vi "FPGAcode2.1.vi"() -> ()   [LabVIEW 2015]
uses:
  Detector_Cluster.ctl
  Limits_In.ctl
  <vilib>/Platform/TimedLoop/XDataNode/timing_clust.ctl
  <vilib>/Platform/TimedLoop/XDataNode/nitl_modes.ctl
  <vilib>/Platform/TimedLoop/XDataNode/wakeup.ctl
  <vilib>/rvi/Emulation/niFpgaSctlEmulationGetInTimedLoop.vi
  <vilib>/rvi/Emulation/niFpgaEmulationReportErrorSimple.vi
  <vilib>/rvi/Emulation/niFpgaGetClockAttributes.vi
  <vilib>/rvi/Emulation/niFpgaCriticalErrorInLSC.vi
  <vilib>/rvi/Emulation/niFpgaProcessEmulError.vi
  <vilib>/rvi/eio/common/nirviEmuTemplateMethod_errors.vi
  <vilib>/Platform/TimedLoop/XDataNode/XDataNode.xnode
  <vilib>/eio/EIONode/EIONode.xnode
  <vilib>/Platform/TimedLoop/XDataNode/XDNodeRunTimeDep.lvlib
panel:
  in  "Limits":T1
  in  "Filter Thresholds":T2
  out "Detector 3 Max Correlations":T2
  out "Detector 3 Correlations":T2
  out "Detector 1 Correlations":T2
  in  "Calibrate":bool
  out "IO Module\\AI 1":i16
  out "IO Module\\AI 0":i16
  out "Del Armed":bool
  out "Armed":bool
  out "Delay":bool
  out "Plates":bool
  in  "Reset One Shot":bool
  in  "One Shot":bool
  in  "Mult1":fxp<+,16,7>
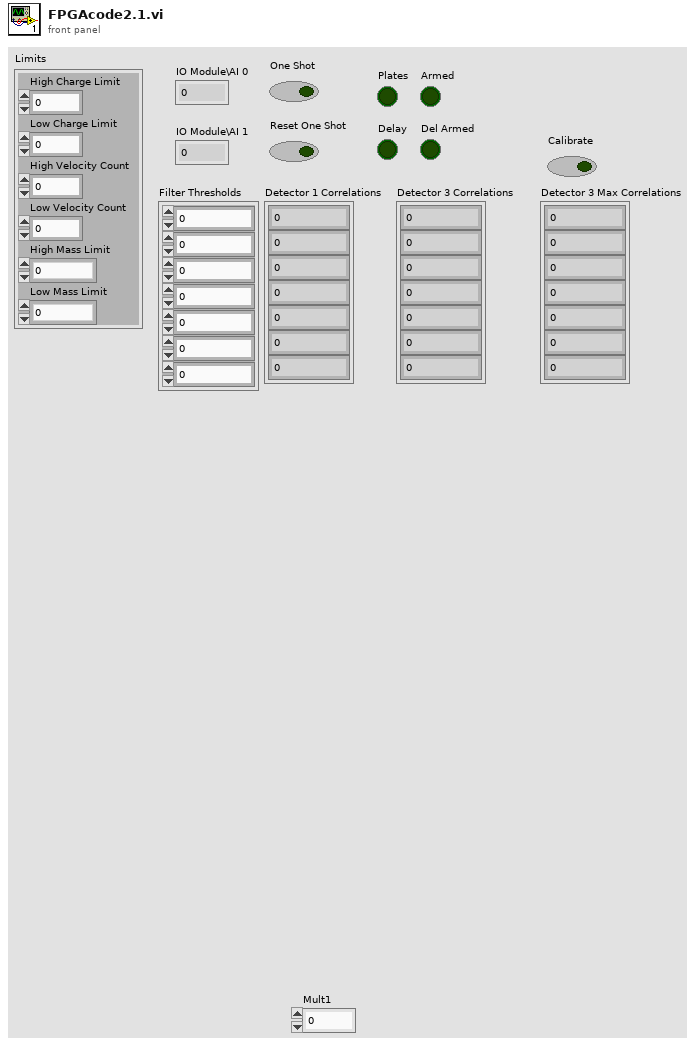
[diagram p1: front panel]
types:
  T1 = typedef "Limits_In.ctl" = cluster{"High Charge Limit":i16, "Low Charge Limit":i16, "High Velocity Count":i32, "Low Velocity Count":i32, "High Mass Limit":i64, "Low Mass Limit":i64}
  T2 = typedef "Detector_Cluster.ctl" = cluster{"1":i32, "2":i32, "3":i32, "4":i32, "5":i32, "6":i32, "7":i32}
  T3 = typedef "XDNodeRunTimeDep.lvlib/timing_clust.ctl" = cluster{"Expected End [f-1]":u64, "Actual End [f-1]":u64, "Finished Late? [f-1]":bool, "Expected End [i-1]":u64, "Actual End [i-1]":u64, "Finished Late? [i-1]":bool, "Expected Start [i]":u64, "Actual Start [i]":u64, "Expected Start [f]":u64, "Actual Start [f]":u64, "Source Name":string, "Structure Name":string, "Period":i64, "Deadline":i64, "Offset":i64, "Start":i64, "Priority":i32, "Timeout":i32, "Mode":T4, "Wakeup Reason":T5, "Error":errorcluster, "Source Type":string, "Secondary Source Type":string, "Global End Time":u64, "Global Start Time":u64, "Frame Duration":u64, "Iteration Duration":u64, "Assigned CPU":i32, "I/O Scan Engine Mode":u32}
  T4 = typedef "XDNodeRunTimeDep.lvlib/nitl_modes.ctl" = enum32{"No Change", "Process missed periods, maintain original phase", "Discard missed periods, maintain original phase", "Process missed periods, ignore original phase", "Discard missed periods, ignore original phase"}
  T5 = typedef "XDNodeRunTimeDep.lvlib/wakeup.ctl" = enum32{"Normal", "Aborted", "Asynchronous wakeup", "Timing source error", "Timed loop error", "Timeout"}
  T6 = cluster{"High Charge Limit":i16, "Low Charge Limit":i16, "Time Out Limit":u32, "High Velocity Count":i32, "Low Velocity Count":i32, "Sampling Rate":fxp<+,30,25>, "High Mass Limit":i64, "Low Mass Limit":i64}
  T7 = cluster{"[0]":i32, "[1]":i32, "[2]":i32, "[3]":i32, "[4]":i32, "[5]":i32, "[6]":i32}
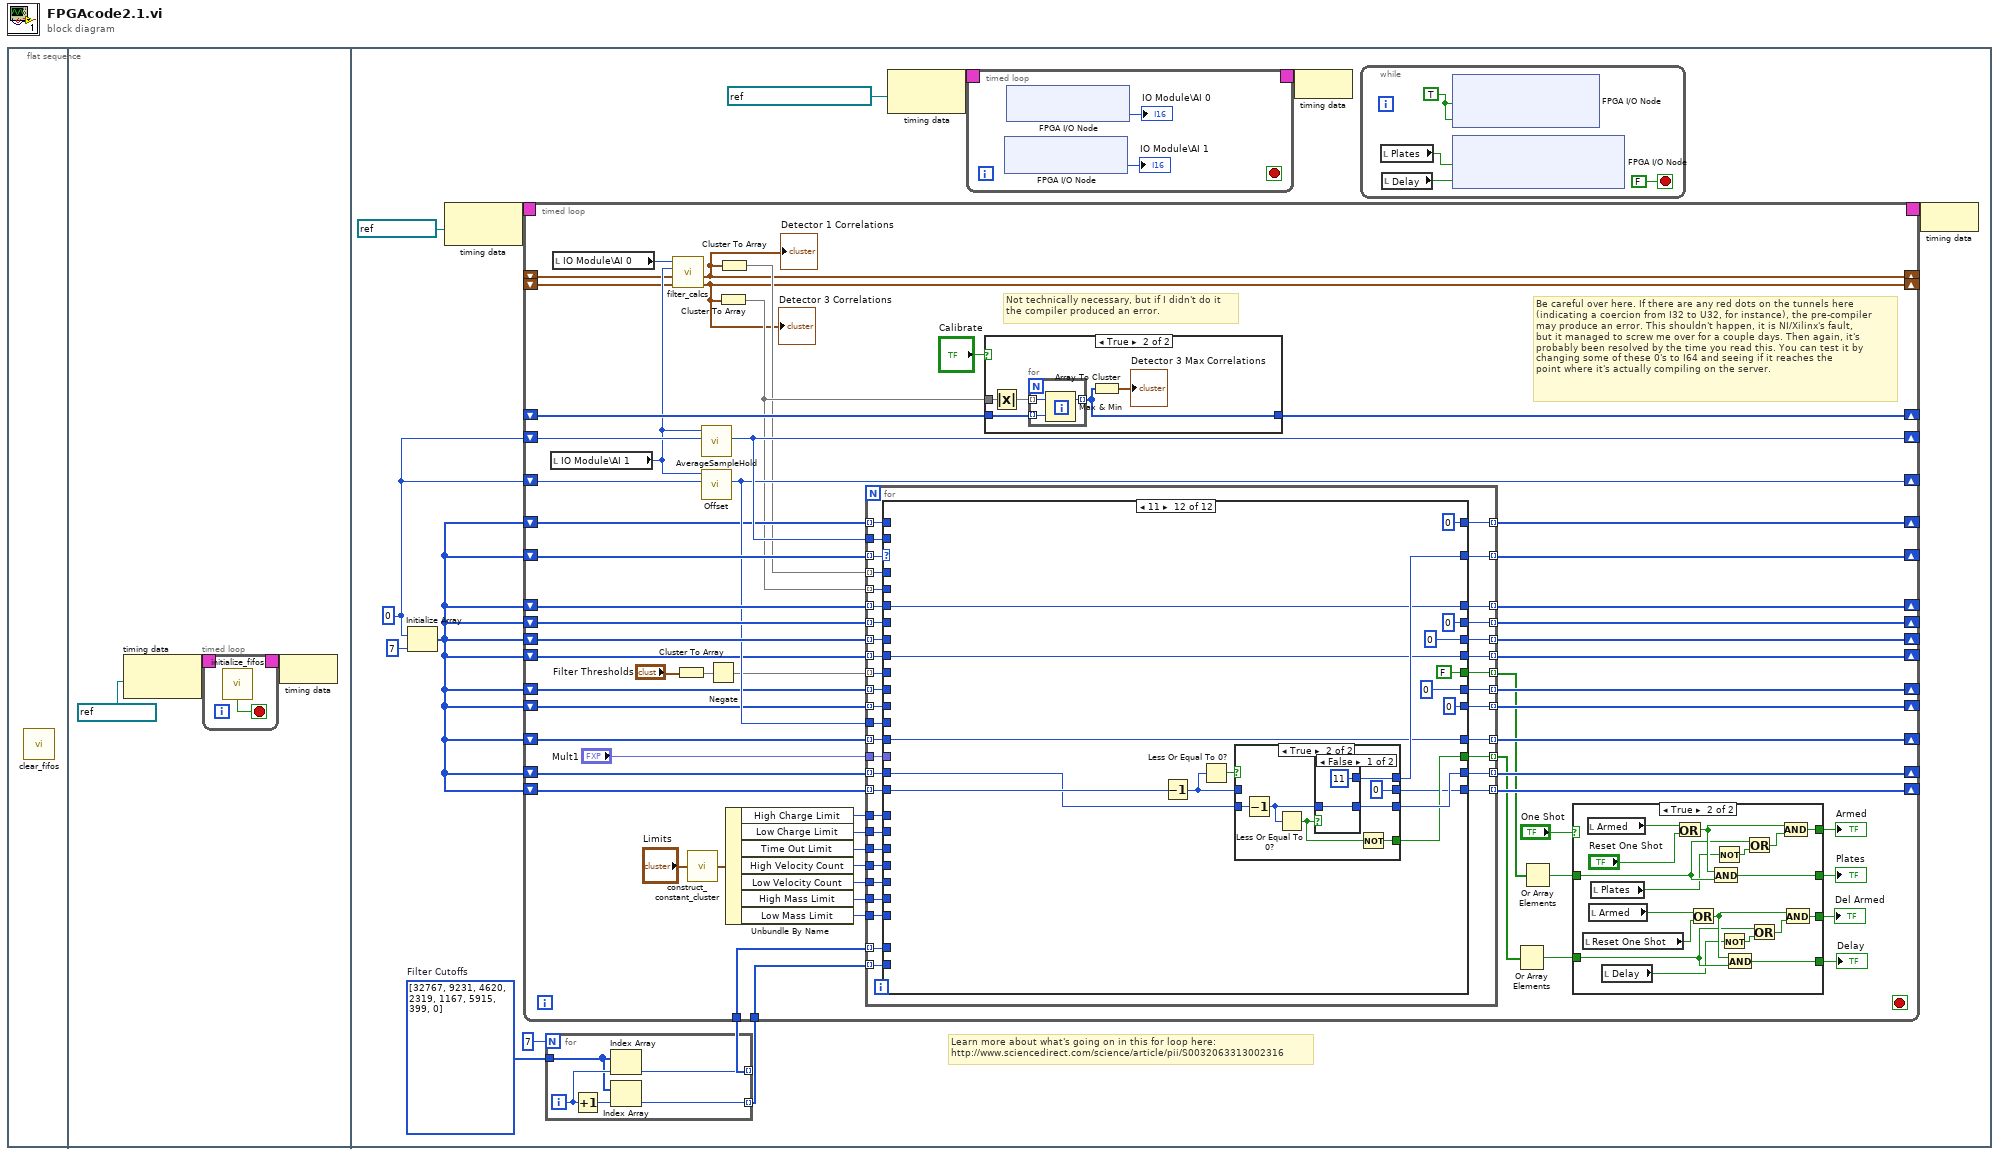
[diagram p0: block diagram]
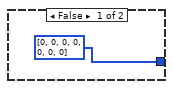
[diagram p2: hidden frame]
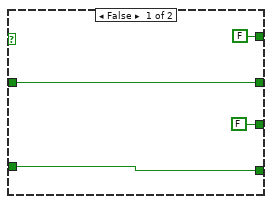
[diagram p3: hidden frame]
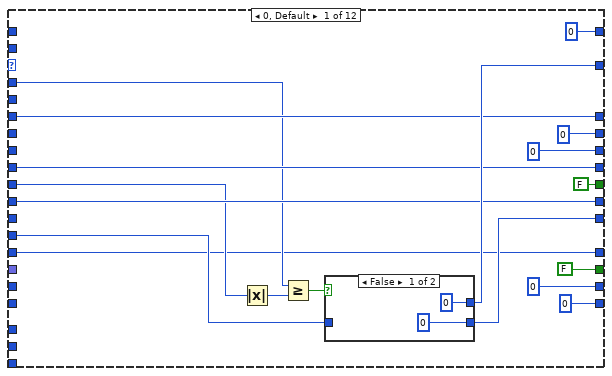
[diagram p4: hidden frame]
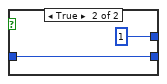
[diagram p5: hidden frame]
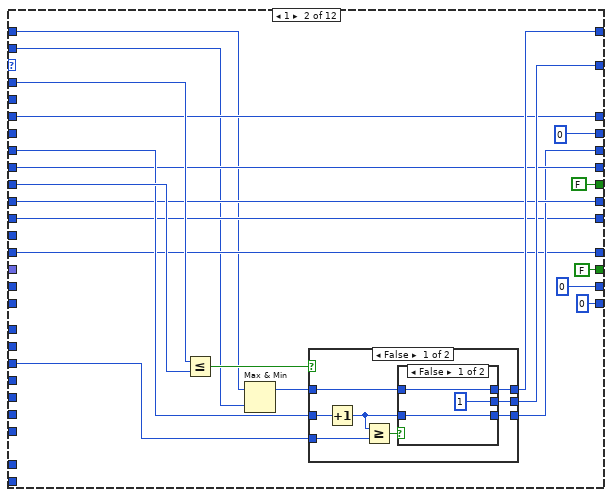
[diagram p6: hidden frame]
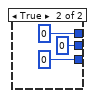
[diagram p7: hidden frame]
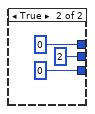
[diagram p8: hidden frame]
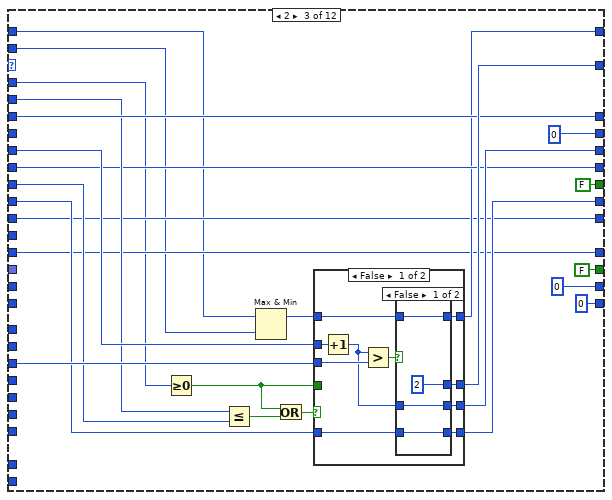
[diagram p9: hidden frame]
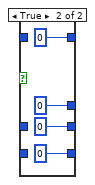
[diagram p10: hidden frame]
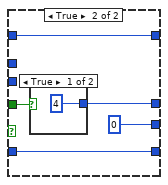
[diagram p11: hidden frame]
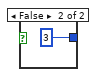
[diagram p12: hidden frame]
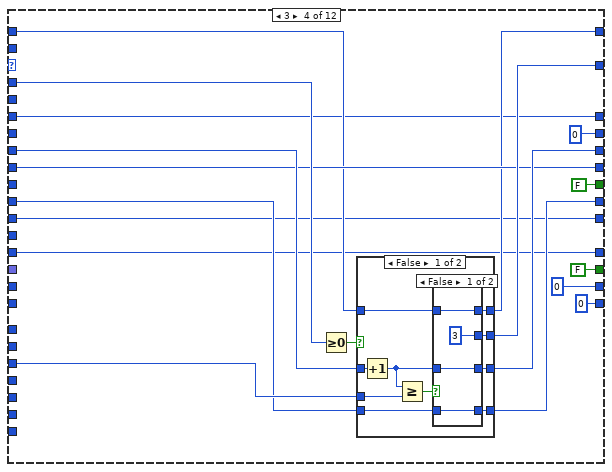
[diagram p13: hidden frame]
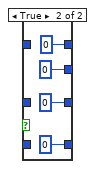
[diagram p14: hidden frame]
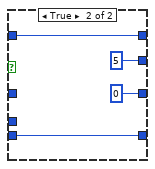
[diagram p15: hidden frame]
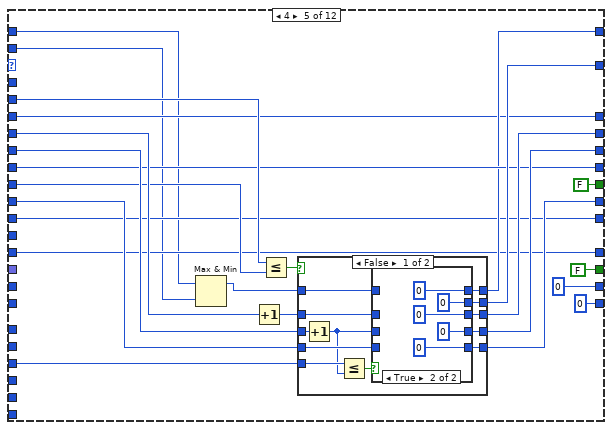
[diagram p16: hidden frame]
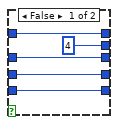
[diagram p17: hidden frame]
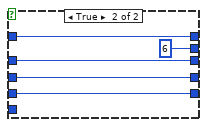
[diagram p18: hidden frame]
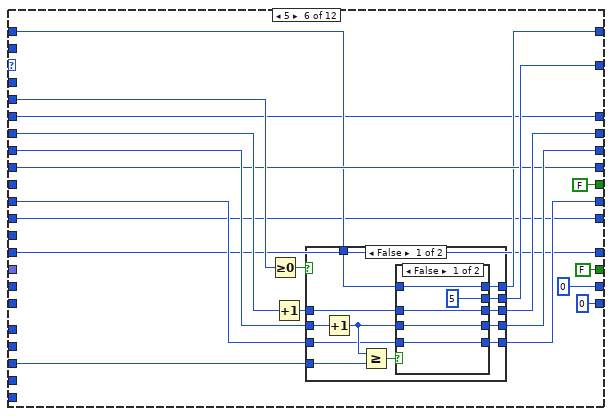
[diagram p19: hidden frame]
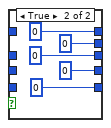
[diagram p20: hidden frame]
diagram:
  n1 = flat-sequence {
    frame #0 {
      n2 = call "clear_fifos.vi"() -> ()  [unwired: 1 in]
    }
    frame #1 {
      n3 = node-c288(refnum<k21> "26.67MHz" ("Source Name")) -> (w3:T3)
      n4 = timed-loop {
        timing: w3 -> [_]
        timing-out: [_] -> w2
        stop <- w4 stop-if-true
        n5 = call "initialize_fifos.vi"() -> ("Output State"=w4:bool)
      }
      n6 = node-c288(w2) -> ()
    }
    frame #2 {
      w11 = 0 ("Output New Average")
      w16 = i16[] [32767, 9231, 4620, 2319, 1167, 5915, 399, 0]  # Filter Cutoffs
      # "Learn more about what's going on in this for loop here:\nhttp://www.sciencedirect.com/science/article/pii/S0032063313002316"
      n7 = Initialize Array(w11, 7 ("dimension size")) -> (w12:i32[])
      n8 = node-c288(refnum<k21> "26.67MHz" ("Source Name")) -> (w23:T3)
      n9 = for {
        N: 7 -> [_]
        tunnel: w16 -> [w26]
        tunnel: [w25] -> w15 mode=indexing
        tunnel: [w24] -> w14 mode=indexing
        i -> [w28]
        n10 = Increment(x=w28) -> (x+1=w27:i32)
        n11 = Index Array(array=w26, index=w28) -> (element=w25:i16)
        n12 = Index Array(array=w26, index=w27) -> (element=w24:i16)
      }
      n13 = timed-loop {
        timing: w23 -> [_]
        timing-out: [_] -> w22
        shift-right: [w100] -> _
        shift-left: w11 -> [w101]
        shift-right: [w98] -> _
        shift-left: w12 -> [w99]
        shift-right: [w84] -> _
        shift-left: w12 -> [w97]
        shift-right: [w95] -> _
        shift-left: w12 -> [w96]
        shift-right: [w93] -> _
        shift-left: w12 -> [w94]
        shift-right: [w83] -> _
        shift-left: w12 -> [w92]
        shift-right: [w82] -> _
        shift-left: w12 -> [w91]
        shift-right: [w78] -> _
        shift-left: w12 -> [w90]
        shift-right: [w88] -> _
        shift-left: w11 -> [w89]
        shift-right: [w81] -> _
        shift-left: w12 -> [w87]
        shift-right: [w80] -> _
        shift-left: w12 -> [w86]
        shift-right: [w79] -> _
        shift-left: w12 -> [w85]
        tunnel: w15 -> [w76]
        tunnel: w14 -> [w75]
        shift-right: [w73] -> _
        shift-left: w12 -> [w74]
        shift-right: [w54] -> _
        shift-left: _ -> [w53]
        shift-right: [w44] -> _
        shift-left: _ -> [w42]
        shift-right: [w43] -> _
        shift-left: _ -> [w41]
        stop <- _ stop-if-true
        # "Be careful over here. If there are any red dots on the tunnels here\n(indicating a coercion from I32 to U32, for instance), the pre-compiler\nmay produce an error. This shouldn't happen, it is NI/Xilinx's fault,\nbut it managed to screw me over for a couple days. Then again, it's\nprobably been resolved by the time you read this. You can test it by\nchanging some of these 0's to I64 and seeing if it reaches the\npoint where it's actually compiling on the server."
        # "Not technically necessary, but if I didn't do it\nthe compiler produced an error."
        n14 = local read "IO Module\\AI 1"() -> (w46:i16)
        n15 = local read "IO Module\\AI 0"() -> (w45:i16)
        n16 = call "filter_calcs.vi"("Detector 3 Correlations In"=w41, "Detector 1 Correlations In"=w42, "Detector 3"=w46, "Detector 1"=w45) -> ("Detector 3 Correlations Out"=w43:T2, "Detector 1 Correlations Out"=w44:T2)  [unwired: 6 in]
        "Detector 1 Correlations" <- w44
        "Detector 3 Correlations" <- w43
        n17 = Cluster To Array(cluster="Filter Thresholds") -> (array=w51:i32[])
        n18 = call "construct_constant_cluster.vi"("Cluster"="Limits") -> ("Limits"=w50:T6)
        n19 = call "AverageSampleHold.vi"("Previous Average"=w101, "Input Value"=w46) -> ("Output New Average"=w100:i32)  [unwired: 9 in]
        n20 = call "Offset.vi"("Previous Average"=w89, "Input Value"=w46) -> ("Output New Average"=w88:i32)  [unwired: 9 in]
        n21 = Negate(x=w51) -> (-x=w56:i32[])
        n22 = Cluster To Array(cluster=w43) -> (array=w48:i32[])
        n23 = Cluster To Array(cluster=w44) -> (array=w47:i32[])
        n24 = Unbundle By Name(w50) -> ("High Charge Limit"=w60:i16, "Low Charge Limit"=w61:i16, "Time Out Limit"=w62:u32, "High Velocity Count"=w63:i32, "Low Velocity Count"=w64:i32, "High Mass Limit"=w65:i64, "Low Mass Limit"=w66:i64)
        n25 = for {
          tunnel: w47 -> [w168] mode=indexing
          tunnel: w48 -> [w167] mode=indexing
          tunnel: w74 -> [w171] mode=indexing
          tunnel: [w154] -> w73 mode=indexing
          tunnel: w99 -> [w169] mode=indexing
          tunnel: [w153] -> w98 mode=indexing
          tunnel: w97 -> [w166] mode=indexing
          tunnel: w96 -> [w133] mode=indexing
          tunnel: [w142] -> w95 mode=indexing
          tunnel: w94 -> [w134] mode=indexing
          tunnel: [w143] -> w93 mode=indexing
          tunnel: w92 -> [w165] mode=indexing
          tunnel: w91 -> [w164] mode=indexing
          tunnel: w90 -> [w158] mode=indexing
          tunnel: w87 -> [w163] mode=indexing
          tunnel: w56 -> [w162] mode=indexing
          tunnel: w86 -> [w161] mode=indexing
          tunnel: w85 -> [w160] mode=indexing
          tunnel: [w152] -> w84 mode=indexing
          tunnel: [w151] -> w83 mode=indexing
          tunnel: [w150] -> w82 mode=indexing
          tunnel: [w149] -> w81 mode=indexing
          tunnel: [w146] -> w80 mode=indexing
          tunnel: [w145] -> w79 mode=indexing
          tunnel: [w144] -> w78 mode=indexing
          tunnel: [w148] -> w72 mode=indexing
          tunnel: [w147] -> w71 mode=indexing
          tunnel: "Mult1" -> [w157]
          tunnel: w100 -> [w170]
          tunnel: w88 -> [w159]
          tunnel: w76 -> [w156] mode=indexing
          tunnel: w75 -> [w155] mode=indexing
          tunnel: w66 -> [w141]
          tunnel: w65 -> [w140]
          tunnel: w64 -> [w139]
          tunnel: w63 -> [w138]
          tunnel: w62 -> [w137]
          tunnel: w61 -> [w136]
          tunnel: w60 -> [w135]
          n26 = case shown="11" w169 {
            tunnel: w168 -> [w182 w214 w235 w296 _ _ _ _ _ _ _ _]
            tunnel: w167 -> [_ _ w248 _ w338 w386 w433 _ _ _ _ _]
            tunnel: w162 -> [w180 w213 w247 _ w337 _ _ _ _ _ _ _]
            tunnel: w165 -> [_ _ _ _ w340 w394 w442 w485 w542 w571 w601 _]
            tunnel: [0 0 0 0 w346 w392 w435 w470 w541 w569 w599 0] -> w151
            tunnel: [w189 w211 w256 w300 w345 w389 w438 w490 w540 w570 w600 w625] -> w153
            tunnel: w166 -> [w186 w207 w249 w287 w330 w378 w434 w491 w516 w555 w597 w616]
            tunnel: w137 -> [_ w209 w255 w299 w343 w387 w439 _ _ _ _ _]
            tunnel: w164 -> [_ w210 w254 w298 w344 w388 w441 _ _ _ _ _]
            tunnel: [u32 0 w202 w253 w297 w342 w390 w437 0 i16 0 ("Timeout Count in") u32 0 ("Timeout Count in") u32 0 u32 0 ("Timeout Count in")] -> w150
            tunnel: w139 -> [_ _ _ _ _ _ _ _ w539 _ _ _]
            tunnel: w138 -> [_ _ _ _ _ _ _ _ w538 _ _ _]
            tunnel: [w186 w207 w249 w287 w330 w378 w434 w492 w516 w555 w597 w616] -> w152
            tunnel: w136 -> [_ _ _ _ _ _ _ _ w537 _ _ _]
            tunnel: w135 -> [_ _ _ _ _ _ _ _ w536 _ _ _]
            tunnel: w161 -> [w185 w204 w246 w294 w336 w381 w432 w488 w535 w567 w595 _]
            tunnel: [w185 w204 w245 w293 w335 w385 w431 w489 w534 w567 w596 0 ("Noise Level")] -> w146
            tunnel: w163 -> [w184 w205 w244 w292 w334 w384 w430 w487 w517 w563 w592 w618]
            tunnel: [w184 w205 w244 w292 w334 w384 w430 w487 w517 w564 w592 w618] -> w149
            tunnel: [0 ("Old Average In") w208 w243 w291 w333 w383 w429 w486 w530 w560 0 ("Old Average In") 0 ("Old Average In")] -> w154
            tunnel: w156 -> [_ _ _ _ _ _ _ w472 _ _ _ _]
            tunnel: w155 -> [_ _ _ _ _ _ _ w471 _ _ _ _]
            tunnel: [FALSE FALSE ("Data") FALSE FALSE FALSE FALSE FALSE FALSE FALSE ("Data") w554 w586 FALSE ("Data")] -> w148
            tunnel: w171 -> [_ w196 w234 w289 w325 w380 w427 w482 w530 w560 _ _]
            tunnel: w170 -> [_ w195 w233 _ w324 _ _ _ _ _ _ _]
            tunnel: w160 -> [_ w201 w241 w288 w331 w379 w426 w481 w531 w559 _ _]
            tunnel: w159 -> [w177 _ _ _ _ _ _ _ _ _ _ _]
            tunnel: [w178 w201 w241 w288 w331 w379 w426 w481 w531 w559 0 ("Offset") 0 ("Offset")] -> w145
            tunnel: [w176 w200 w240 w286 w329 w377 w425 w480 w518 w565 w590 w623] -> w144
            tunnel: w158 -> [w176 w200 w240 w286 w329 w377 w425 w480 w518 w566 w590 w623]
            tunnel: w140 -> [_ _ _ _ _ _ _ _ w529 _ _ _]
            tunnel: w141 -> [_ _ _ _ _ _ _ _ w528 _ _ _]
            tunnel: w133 -> [_ _ _ _ _ _ _ _ w524 w558 w589 w614]
            tunnel: [0 0 0 0 0 0 0 w476 w523 w556 w584 w611] -> w142
            tunnel: [FALSE FALSE FALSE FALSE FALSE FALSE FALSE FALSE FALSE w553 w585 w615] -> w147
            tunnel: [0 0 0 0 0 0 0 0 0 0 w588 w624] -> w143
            tunnel: w134 -> [_ _ _ _ _ _ _ _ _ _ _ w612]
            tunnel: w157 -> [_ _ _ _ _ _ _ w475 _ _ _ _]
            frame 0, Default {
              n27 = Absolute Value(x=w180) -> (abs(x)=w179:i32)
              n28 = Greater Or Equal?(x=w182, y=w179) -> (x >= y?=w187:bool)
              n29 = case shown="False" w187 {
                tunnel: [i8 0 i8 1] -> w189
                tunnel: [0 w192] -> w178
                tunnel: w177 -> [_ w192]
                frame False {
                }
                frame True {
                }
              }
            }
            frame 1 {
              n30 = Less Or Equal?(x=w214, y=w213) -> (x <= y?=w212:bool)
              n31 = Max & Min(x=w196, y=w195) -> (max(x,y)=w194:i32)  [unwired: 1 out]
              n32 = case shown="False" w212 {
                tunnel: [w220 i8 2] -> w211
                tunnel: w210 -> [w217 _]
                tunnel: w209 -> [w222 _]
                tunnel: w194 -> [w219 _]
                tunnel: [w218 0 ("New Average")] -> w208
                tunnel: [w215 u32 0] -> w202
                frame False {
                  n33 = Increment(x=w217) -> (x+1=w216:u32)
                  n34 = Greater Or Equal?(x=w216, y=w222) -> (x >= y?=w221:bool)
                  n35 = case shown="False" w221 {
                    tunnel: [i8 1 i8 0] -> w220
                    tunnel: w219 -> [w225 _]
                    tunnel: [w225 0 ("New Average")] -> w218
                    tunnel: w216 -> [w223 _]
                    tunnel: [w223 u32 0] -> w215
                    frame False {
                    }
                    frame True {
                    }
                  }
                }
                frame True {
                }
              }
            }
            frame 2 {
              n36 = Greater Or Equal To 0?(x=w235) -> (x >= 0?=w251:bool)
              n37 = Less Or Equal?(x=w248, y=w247) -> (x <= y?=w250:bool)
              n38 = Max & Min(x=w234, y=w233) -> (max(x,y)=w232:i32)  [unwired: 1 out]
              n39 = Or(x=w251, y=w250) -> (x .or. y?=w252:bool)
              n40 = case shown="False" w252 {
                tunnel: [w264 w275] -> w256
                tunnel: w255 -> [w266 _]
                tunnel: w254 -> [w263 _]
                tunnel: [w262 u32 0] -> w253
                tunnel: w251 -> [_ w276]
                tunnel: w246 -> [w261 w278]
                tunnel: [w260 w278] -> w245
                tunnel: [w259 w279] -> w243
                tunnel: w232 -> [w257 w279]
                frame False {
                  n41 = Increment(x=w263) -> (x+1=w258:u32)
                  n42 = Greater?(x=w258, y=w266) -> (0:w265:bool)
                  n43 = case shown="False" w265 {
                    tunnel: [i8 2 i8 0 ("Old Average In")] -> w264
                    tunnel: w258 -> [w267 _]
                    tunnel: [w267 u32 0 ("Old Average In")] -> w262
                    tunnel: w261 -> [w269 _]
                    tunnel: [w269 0 ("Old Average In")] -> w260
                    tunnel: [w268 0 ("Old Average In")] -> w259
                    tunnel: w257 -> [w268 _]
                    frame False {
                    }
                    frame True {
                    }
                  }
                }
                frame True {
                  n44 = case shown="True" w276 {
                    tunnel: [i8 4 i8 3] -> w275
                    frame True {
                    }
                    frame False {
                    }
                  }
                }
              }
            }
            frame 3 {
              n45 = Greater Or Equal To 0?(x=w296) -> (x >= 0?=w295:bool)
              n46 = case shown="False" w295 {
                tunnel: [w309 i8 5] -> w300
                tunnel: w299 -> [w308 _]
                tunnel: w298 -> [w306 _]
                tunnel: [w307 u32 0] -> w297
                tunnel: w294 -> [w305 w320]
                tunnel: [w304 w320] -> w293
                tunnel: [w303 w319] -> w291
                tunnel: w289 -> [w302 w319]
                frame False {
                  n47 = Increment(x=w306) -> (x+1=w301:u32)
                  n48 = Greater Or Equal?(x=w301, y=w308) -> (x >= y?=w310:bool)
                  n49 = case shown="False" w310 {
                    tunnel: [i8 3 i8 0] -> w309
                    tunnel: w301 -> [w311 _]
                    tunnel: [w311 u32 0] -> w307
                    tunnel: w305 -> [w313 _]
                    tunnel: [w313 0 ("High Correlation In")] -> w304
                    tunnel: [w312 0 ("Old Average In")] -> w303
                    tunnel: w302 -> [w312 _]
                    frame False {
                    }
                    frame True {
                    }
                  }
                }
                frame True {
                }
              }
            }
            frame 4 {
              n50 = Max & Min(x=w325, y=w324) -> (max(x,y)=w323:i32)  [unwired: 1 out]
              n51 = Increment(x=w340) -> (x+1=w339:i32)
              n52 = Less Or Equal?(x=w338, y=w337) -> (x <= y?=w341:bool)
              n53 = case shown="False" w341 {
                tunnel: w339 -> [w354 w373]
                tunnel: [w353 w373] -> w346
                tunnel: [w356 i8 6] -> w345
                tunnel: w344 -> [w352 w369]
                tunnel: w343 -> [w358 _]
                tunnel: [w355 w369] -> w342
                tunnel: w336 -> [w351 w371]
                tunnel: [w350 w371] -> w335
                tunnel: [w349 w370] -> w333
                tunnel: w323 -> [w348 w370]
                frame False {
                  n54 = Increment(x=w352) -> (x+1=w347:u32)
                  n55 = Less Or Equal?(x=w358, y=w347) -> (x <= y?=w357:bool)
                  n56 = case shown="True" w357 {
                    tunnel: [i8 4 i8 0] -> w356
                    tunnel: w347 -> [w362 _]
                    tunnel: [w362 u32 0] -> w355
                    tunnel: w354 -> [w361 _]
                    tunnel: [w361 0] -> w353
                    tunnel: w351 -> [w360 _]
                    tunnel: [w360 0 ("High Correlation In")] -> w350
                    tunnel: [w359 0 ("Old Average In")] -> w349
                    tunnel: w348 -> [w359 _]
                    frame False {
                    }
                    frame True {
                    }
                  }
                }
                frame True {
                }
              }
            }
            frame 5 {
              n57 = Greater Or Equal To 0?(x=w386) -> (x >= 0?=w393:bool)
              n58 = Increment(x=w394) -> (x+1=w391:i32)
              n59 = case shown="False" w393 {
                tunnel: [w399 w421] -> w392
                tunnel: w391 -> [w400 w421]
                tunnel: [w402 u32 0] -> w390
                tunnel: [w404 i8 7] -> w389
                tunnel: w388 -> [w406 _]
                tunnel: w387 -> [w401 _]
                tunnel: w381 -> [w398 w418]
                tunnel: [w397 w418] -> w385
                tunnel: [w396 w417] -> w383
                tunnel: w380 -> [w395 w417]
                frame False {
                  n60 = Increment(x=w406) -> (x+1=w403:u32)
                  n61 = Greater Or Equal?(x=w403, y=w401) -> (x >= y?=w405:bool)
                  n62 = case shown="False" w405 {
                    tunnel: [i8 5 i8 0] -> w404
                    tunnel: w403 -> [w410 _]
                    tunnel: [w410 u32 0] -> w402
                    tunnel: w400 -> [w409 _]
                    tunnel: [w409 0] -> w399
                    tunnel: w398 -> [w408 _]
                    tunnel: [w408 0 ("High Correlation In")] -> w397
                    tunnel: [w407 0 ("Old Average In")] -> w396
                    tunnel: w395 -> [w407 _]
                    frame False {
                    }
                    frame True {
                    }
                  }
                }
                frame True {
                }
              }
            }
            frame 6 {
              n63 = Increment(x=w441) -> (x+1=w440:u32)
              n64 = Greater Or Equal To 0?(x=w433) -> (x >= 0?=w443:bool)
              n65 = Increment(x=w442) -> (x+1=w436:i32)
              n66 = case shown="False" w443 {
                tunnel: w440 -> [w450 _]
                tunnel: w439 -> [w454 _]
                tunnel: [w452 i8 7] -> w438
                tunnel: [w451 u32 0] -> w437
                tunnel: w436 -> [w449 w467]
                tunnel: [w448 w467] -> w435
                tunnel: w432 -> [w446 w466]
                tunnel: [w447 w466] -> w431
                tunnel: [w445 w465] -> w429
                tunnel: w427 -> [w444 w465]
                frame False {
                  n67 = Greater Or Equal?(x=w450, y=w454) -> (x >= y?=w453:bool)
                  n68 = case shown="False" w453 {
                    tunnel: [i8 6 i8 0] -> w452
                    tunnel: [w458 u32 0] -> w451
                    tunnel: w450 -> [w458 _]
                    tunnel: w449 -> [w457 _]
                    tunnel: [w457 0] -> w448
                    tunnel: [w456 0 ("High Correlation In")] -> w447
                    tunnel: w446 -> [w456 _]
                    tunnel: [w455 0 ("Old Average In")] -> w445
                    tunnel: w444 -> [w455 _]
                    frame False {
                    }
                    frame True {
                    }
                  }
                }
                frame True {
                }
              }
            }
            frame 7 {
              n69 = Less?(x=w485, y=w472) -> (x < y?=w474:bool)
              n70 = Greater Or Equal?(x=w485, y=w471) -> (x >= y?=w473:bool)
              n71 = And(x=w474, y=w473) -> (x .and. y?=w484:bool)
              n72 = case shown="False" w484 {
                tunnel: [0 w502] -> w470
                tunnel: w485 -> [_ w501]
                tunnel: [w498 w501] -> w492
                tunnel: w491 -> [w498 _]
                tunnel: [i8 0 i8 8] -> w490
                tunnel: [0 ("High Correlation In") w506] -> w489
                tunnel: w488 -> [_ w506]
                tunnel: [0 ("Old Average In") w505] -> w486
                tunnel: w482 -> [_ w505]
                frame False {
                }
                frame True {
                  n73 = Multiply(x=w501, y=fxp<+,6,1> 1.40625) -> (x*y=w500:fxp<+/-,38,33>)
                  n74 = To Long Integer(number=w500) -> (32bit integer=w499:i32)
                  n75 = Subtract(x=w499, y=19) -> (x-y=w502:i32)
                }
              }
              n76 = Multiply(x=w470, y=w475) -> (x*y=w478:fxp<+/-,48,39>)
              n77 = To Long Integer(number=w478) -> (32bit integer=w476:i32)
            }
            frame 8 {
              n78 = Square(x=w516) -> (x^2=w512:i32)
              n79 = Subtract(x=w531, y=w530) -> (x-y=w533:i32)
              n80 = To Quad Integer(1:w512) -> (0:w525:i64)
              n81 = Absolute Value(x=w533) -> (abs(x)=w511:i32)
              n82 = To Quad Integer(1:w511) -> (0:w526:i64)
              n83 = Greater Or Equal?(x=w536, y=w511) -> (x >= y?=w515:bool)
              n84 = Less Or Equal?(x=w537, y=w511) -> (x <= y?=w514:bool)
              n85 = Multiply(x=w526, y=w525) -> (x*y=w527:i64)
              n86 = Greater Or Equal?(x=w516, y=w538) -> (x >= y?=w513:bool)
              n87 = Less Or Equal?(x=w516, y=w539) -> (x <= y?=w510:bool)
              n88 = Less Or Equal?(x=w527, y=w529) -> (x <= y?=w508:bool)
              n89 = Greater Or Equal?(x=w527, y=w528) -> (x >= y?=w509:bool)
              n90 = Compound Arithmetic op=AND(w515, w514, w513, w510, w508, w509) -> (w532:bool)
              n91 = case shown="True" w532 {
                tunnel: w542 -> [_ w552]
                tunnel: [0 w550] -> w541
                tunnel: [i8 0 i8 9] -> w540
                tunnel: w535 -> [_ w551]
                tunnel: [0 ("High Correlation In") w551] -> w534
                tunnel: w524 -> [_ w548]
                tunnel: [0 w547] -> w523
                frame False {
                }
                frame True {
                  n92 = Decrement(x=w552) -> (x-1=w550:i32)
                  n93 = Decrement(x=w548) -> (x-1=w547:i32)
                }
              }
            }
            frame 9 {
              n94 = Decrement(x=w571) -> (x-1=w572:i32)
              n95 = Subtract(x=w559, y=w560) -> (x-y=w562:i32)
              n96 = Less Or Equal To 0?(x=w572) -> (x <= 0?=w554:bool)
              n97 = Absolute Value(x=w562) -> (abs(x)=w561:i32)
              n98 = case shown="True" w554 {
                tunnel: [i8 9 i8 10] -> w570
                tunnel: [w576 w582] -> w569
                tunnel: w555 -> [_ w580]
                tunnel: w572 -> [w576 _]
                tunnel: w566 -> [w574 _]
                tunnel: [w574 w580] -> w565
                tunnel: [w573 w579] -> w564
                tunnel: w563 -> [w573 _]
                tunnel: w561 -> [_ w579]
                frame False {
                }
                frame True {
                  n99 = To Fixed-Point(number=w580) -> (fixed-point=w577:fxp<+/-,32,32>)  [unwired: 1 in]
                  n100 = Multiply(x=fxp<+,2,1> 1.5, y=w577) -> (x*y=w583:fxp<+/-,34,33>)
                  n101 = To Long Integer(number=w583) -> (32bit integer=w582:i32)
                }
              }
              n102 = Decrement(x=w558) -> (x-1=w556:i32)
              n103 = Less Or Equal To 0?(x=w556) -> (x <= 0?=w553:bool)
            }
            frame 10 {
              n104 = Decrement(x=w601) -> (x-1=w598:i32)
              n105 = Less Or Equal To 0?(x=w598) -> (x <= 0?=w587:bool)
              n106 = case shown="False" w587 {
                tunnel: [w604 0] -> w599
                tunnel: [i8 10 i8 11] -> w600
                tunnel: w598 -> [w604 _]
                tunnel: w595 -> [w603 _]
                tunnel: [w603 0 ("Noise Level")] -> w596
                tunnel: [0 550] -> w588
                frame False {
                }
                frame True {
                }
              }
              n107 = Decrement(x=w589) -> (x-1=w584:i32)
              n108 = Not(x=w587) -> (.not. x?=w586:bool)
              n109 = Less Or Equal To 0?(x=w584) -> (x <= 0?=w585:bool)
            }
            frame 11 {
              n110 = Decrement(x=w614) -> (x-1=w610:i32)
              n111 = Less Or Equal To 0?(x=w610) -> (x <= 0?=w613:bool)
              n112 = case shown="True" w613 {
                tunnel: [FALSE w631] -> w615
                tunnel: [i8 11 w636] -> w625
                tunnel: w612 -> [w629 w637]
                tunnel: [w629 w635] -> w624
                tunnel: [w627 0] -> w611
                tunnel: w610 -> [w627 _]
                frame False {
                }
                frame True {
                  n113 = Decrement(x=w637) -> (x-1=w634:i32)
                  n114 = Less Or Equal To 0?(x=w634) -> (x <= 0?=w632:bool)
                  n115 = case shown="False" w632 {
                    tunnel: [i8 11 i8 0] -> w636
                    tunnel: [w638 0] -> w635
                    tunnel: w634 -> [w638 _]
                    frame False {
                    }
                    frame True {
                    }
                  }
                  n116 = Not(x=w632) -> (.not. x?=w631:bool)
                }
              }
            }
          }
        }
        n117 = case shown="True" "Calibrate" {
          tunnel: w48 -> [_ w106]
          tunnel: w53 -> [_ w105]
          tunnel: [i16[] [0, 0, 0, 0, 0, 0, 0] w104] -> w54
          frame False {
          }
          frame True {
            n118 = Absolute Value(x=w106) -> (abs(x)=w103:i32[])
            n119 = for {
              tunnel: w105 -> [w110] mode=indexing
              tunnel: [w109] -> w104 mode=indexing
              tunnel: w103 -> [w108] mode=indexing
              n120 = Max & Min(x=w108, y=w110) -> (max(x,y)=w109:i32)  [unwired: 1 out]
            }
            n121 = Array To Cluster(array=w104) -> (cluster=→"Detector 3 Max Correlations":T7)
          }
        }
        n122 = Or Array Elements(Boolean array=w71) -> (logical OR=w59:bool)
        n123 = Or Array Elements(Boolean array=w72) -> (logical OR=w70:bool)
        n124 = case shown="True" "One Shot" {
          tunnel: [w114 w128] -> w77
          tunnel: w70 -> [w114 w125]
          tunnel: [FALSE w130] -> w69
          tunnel: [FALSE w118] -> w58
          tunnel: w59 -> [w112 w117]
          tunnel: [w112 w116] -> w57
          frame False {
          }
          frame True {
            n125 = local read "Reset One Shot"() -> (w123:bool)
            n126 = local read "Armed"() -> (w132:bool)
            n127 = local read "Armed"() -> (w119:bool)
            n128 = local read "Plates"() -> (w124:bool)
            n129 = local read "Delay"() -> (w115:bool)
            n130 = Or(x=w132, y="Reset One Shot") -> (x .or. y?=w129:bool)
            n131 = Or(x=w119, y=w123) -> (x .or. y?=w120:bool)
            n132 = And(x=w129, y=w125) -> (x .and. y?=w128:bool)
            n133 = Not(x=w124) -> (.not. x?=w126:bool)
            n134 = Not(x=w115) -> (.not. x?=w122:bool)
            n135 = And(x=w120, y=w117) -> (x .and. y?=w116:bool)
            n136 = Or(x=w125, y=w126) -> (x .or. y?=w127:bool)
            n137 = Or(x=w117, y=w122) -> (x .or. y?=w121:bool)
            n138 = And(x=w129, y=w127) -> (x .and. y?=w130:bool)
            n139 = And(x=w120, y=w121) -> (x .and. y?=w118:bool)
          }
        }
        "Plates" <- w77
        "Delay" <- w57
        "Armed" <- w69
        "Del Armed" <- w58
      }
      n140 = node-c288(refnum<k21> "IO Module\\Data Clock" ("Source Name")) -> (w20:T3)
      n141 = timed-loop {
        timing: w20 -> [_]
        timing-out: [_] -> w19
        stop <- _ stop-if-true
        n142 = xnode "FPGA I/O Node"() -> ("IO Module\\AI 1"=→"IO Module\\AI 1":i16)  [unwired: 1 in, 1 out]
        n143 = xnode "FPGA I/O Node"() -> ("IO Module\\AI 0"=→"IO Module\\AI 0":i16)  [unwired: 1 in, 1 out]
      }
      n144 = node-c288(w19) -> ()
      n145 = while {
        stop <- FALSE stop-if-true
        w40 = TRUE ("IO Module\\PFI Enable")
        n146 = local read "Plates"() -> (w38:bool)
        n147 = local read "Delay"() -> (w37:bool)
        n148 = xnode "FPGA I/O Node"("IO Module\\PFI 0 WE"=w40, "IO Module\\PFI 1 WE"=w40) -> ()  [unwired: 2 in, 2 out]
        n149 = xnode "FPGA I/O Node"("IO Module\\PFI 0 Wr Data"=w38, "IO Module\\PFI 1 Wr Data"=w37) -> ()  [unwired: 2 in, 2 out]
      }
      n150 = node-c288(w22) -> ()
    }
  }
